vi "Place Left Gear.vi"(8 "error in":errorcluster) -> (0 "error out":errorcluster)   [LabVIEW 2016]
uses:
  Refname/Motors.ctl
  Refname/Refname to String (Motors).vi
panel:
  in  "Distance(in) Backwards":dbl format="%#_13g"
  in  "Distance (in) Forward":dbl format="%#_13g"
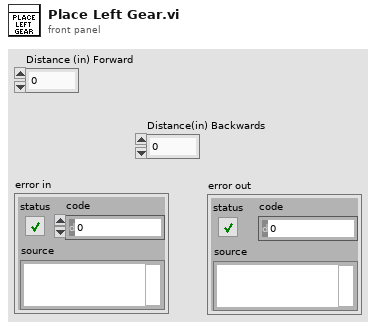
[diagram p1: front panel]
types:
  T1 = typedef "Motors.ctl" = enum16{"Wheel 1", "Swerve 1", "Wheel 2", "Swerve 2", "Wheel 3", "Swerve 3", "Wheel 4", "Swerve 4"}
  T2 = typedef "WPI_MotorControlDeviceRef.ctl" = cluster{"DeviceStatus":errorcluster, "Type":T3, "PWM":cluster{"PWM Channel":T4, "DeadBand":T5}, "CAN":cluster{"Device Number":u8, "SetOutput VI Ref":variant, "GetOutput VI Ref":variant, "Enable VI Ref":variant, "Disable VI Ref":variant, "Data":variant}, "Invert":bool}
  T3 = typedef "WPI_MotorControlType.ctl" = enum16{"PWM", "CAN"}
  T4 = typedef "FPGA_DIOPWMChannel.ctl" = enum8{"PWM 0", "PWM 1", "PWM 2", "PWM 3", "PWM 4", "PWM 5", "PWM 6", "PWM 7", "PWM 8", "PWM 9", "PWM MXP 0", "PWM MXP 1", "PWM MXP 2", "PWM MXP 3", "PWM MXP 4", "PWM MXP 5", "PWM MXP 6", "PWM MXP 7", "PWM MXP 8", "PWM MXP 9", "Invalid"}
  T5 = typedef "WPI_PWMDeadband.ctl" = cluster{"Name":string, "maxPositivePwm":i32, "minPositivePwm":i32, "centerPwm":i32, "maxNegativePwm":i32, "minNegativePwm":i32, "angularRange":u16}
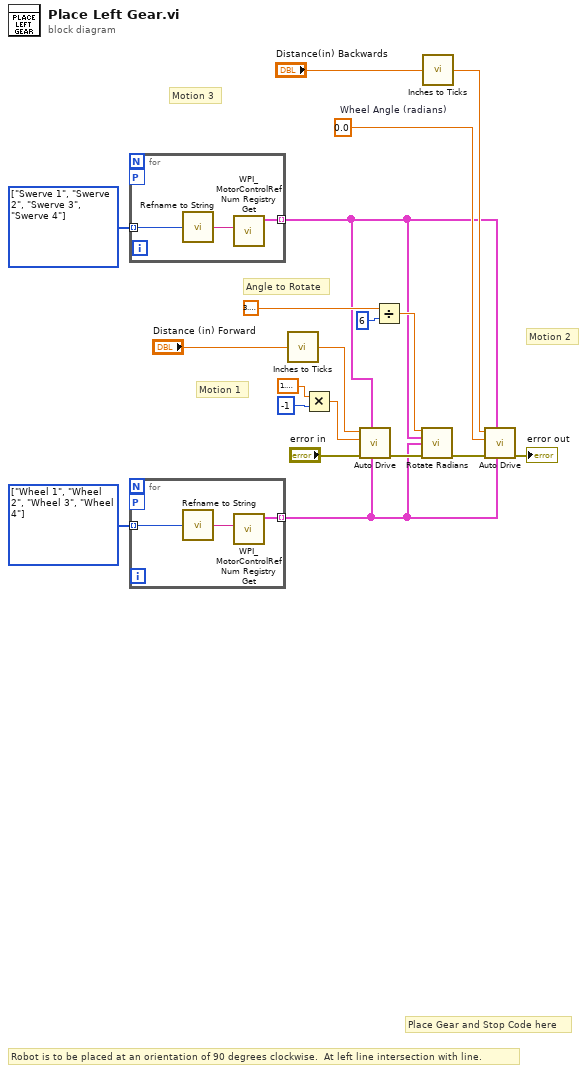
[diagram p0: block diagram]
diagram:
  w3 = T1[] [enum."Swerve 1", enum."Swerve 2", enum."Swerve 3", enum."Swerve 4"] items=["Wheel 1", "Swerve 1", "Wheel 2", "Swerve 2", "Wheel 3", "Swerve 3", "Wheel 4", "Swerve 4"]
  w4 = T1[] [enum."Wheel 1", enum."Wheel 2", enum."Wheel 3", enum."Wheel 4"] items=["Wheel 1", "Swerve 1", "Wheel 2", "Swerve 2", "Wheel 3", "Swerve 3", "Wheel 4", "Swerve 4"]
  w7 = 0.0  # Wheel Angle (radians)
  # "Robot is to be placed at an orientation of 90 degrees clockwise.  At left line intersection with line."
  # "Place Gear and Stop Code here"
  # "Motion 3"
  # "Motion 2"
  # "Motion 1"
  # "Angle to Rotate"
  n1 = for {
    workers-P: _ -> [_]
    tunnel: w3 -> [w22] mode=indexing
    tunnel: [w20] -> w2 mode=indexing
    n2 = call-poly "Refname to String.vi"("Enum"=w22) -> ("String"=w21:string)
    n3 = call <vilib>:"WPI_MotorControlRefNum Registry Get.vi"("refnum name"=w21) -> ("MotorControlDevRef"=w20:T2)  [unwired: 9 in, 1 out]
  }
  n4 = for {
    workers-P: _ -> [_]
    tunnel: w4 -> [w25] mode=indexing
    tunnel: [w23] -> w1 mode=indexing
    n5 = call-poly "Refname to String.vi"("Enum"=w25) -> ("String"=w24:string)
    n6 = call <vilib>:"WPI_MotorControlRefNum Registry Get.vi"("refnum name"=w24) -> ("MotorControlDevRef"=w23:T2)  [unwired: 9 in, 1 out]
  }
  n7 = call "Inches to Ticks.vi"("Inches"="Distance (in) Forward") -> ("Ticks"=w10:dbl)
  n8 = Multiply(x=1.5707963267948966, y=-1) -> (x*y=w14:dbl)
  n9 = call "Auto Drive.vi"("Wheel DevRef"=w1, "Swerve DevRef"=w2, "error in"="error in", "Drive Angle"=w14, "Ticks(Distance)"=w10) -> ("error out"=w12:errorcluster)  [unwired: 6 in]
  n10 = Divide(x=3.141592653589793, y=6) -> (x/y=w16:dbl)
  n11 = call "Rotate Radians.vi"("Radians to turn(Direction)"=w16, "Swerve DevRef"=w2, "Wheel DevRef"=w1, "error in"=w12) -> ("error constant"=w9:errorcluster)  [unwired: 11 in]
  n12 = call "Inches to Ticks.vi"("Inches"="Distance(in) Backwards") -> ("Ticks"=w5:dbl)
  n13 = call "Auto Drive.vi"("Wheel DevRef"=w1, "Swerve DevRef"=w2, "error in"=w9, "Drive Angle"=w7, "Ticks(Distance)"=w5) -> ("error out"=→"error out":errorcluster)  [unwired: 6 in]
